vi "Configure Filter.vi"(0 "VISA resource name":refnum<visa-resource-name>, 1 "Scan List (Empty)":string, 5 "Filter Type (0:Off)":u16(ring) items=["Off", "Moving", "Repeat"], 7 "Filter Window (%) (0.1)":dbl=0.1, 9 "Filter Count (10)":i32=10, 11 "error in (no error)":errorcluster) -> (4 "VISA resource name out":refnum<visa-resource-name>, 15 "error out":errorcluster)   [LabVIEW 2020, in "Keithley 27XX.lvlib"]
doc: "This VI configures the filter attributes for the current measurement function.\nFiltering allows you to stabilize noisy measurements. \n\nThe filter setup is \"remembered\" and can be unique for each measurement function. When you change functions , the instrument will return to the last filter setup for that function.\n\nNote: \n(1) Configure Measurement.vi must be called <B>before</B> setting the filter.\n\n(2) This VI should not be used with the measurement functions Frequency, Period, or Continuity."
uses:
  <instrlib>/Keithley 27XX/Keithley 27XX.lvlib
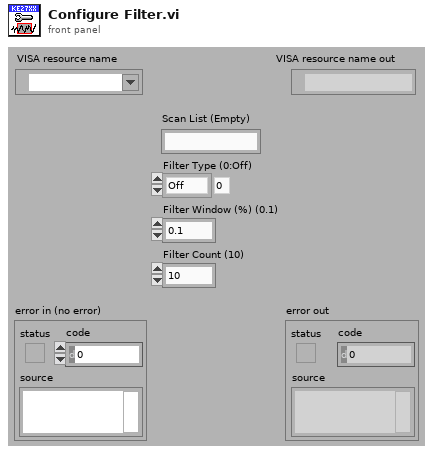
[diagram p1: front panel]
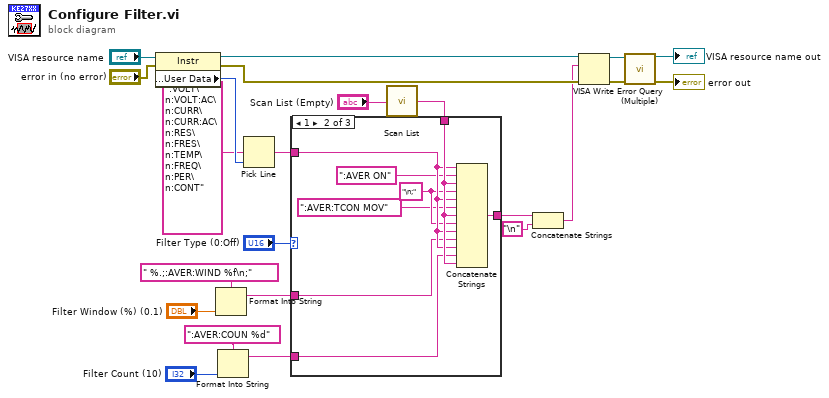
[diagram p0: block diagram]
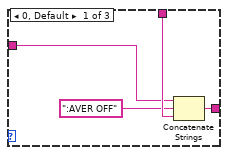
[diagram p2: hidden frame]
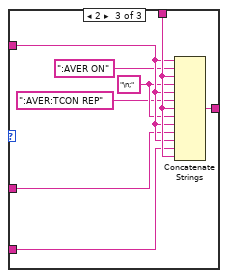
[diagram p3: hidden frame]
diagram:
  n1 = property on="Property Node" class="Instr"(reference="VISA resource name", error in="error in (no error)") -> (reference out=w19:refnum<visa-resource-name>, error out=w18:errorcluster, "General Settings:User Data"=w23:u32)
  n2 = Format Into String(format string=" %.;:AVER:WIND %f\n;", "Filter Window (%) (0.1)") -> (resulting string=w11:string)  [unwired: 2 in, 1 out]
  n3 = Format Into String(format string=":AVER:COUN %d", "Filter Count (10)") -> (resulting string=w9:string)  [unwired: 2 in, 1 out]
  n4 = Pick Line(multi-line string=":VOLT\n:VOLT:AC\n:CURR\n:CURR:AC\n:RES\n:FRES\n:TEMP\n:FREQ\n:PER\n:CONT", line index=w23) -> (output string=w20:string)  [unwired: 1 in]
  n5 = call <instrlib>:"Scan List.vi"("Scan List (Empty)"="Scan List (Empty)") -> ("Scan List Out"=w14:string)  [unwired: 14 in]
  n6 = case shown="1" "Filter Type (0:Off)" {
    tunnel: w20 -> [w25 w33 w41]
    tunnel: w14 -> [w26 w34 w42]
    tunnel: w11 -> [_ w31 w37]
    tunnel: w9 -> [_ w30 w36]
    tunnel: [w27 w35 w43] -> w2
    frame 0, Default {
      n7 = Concatenate Strings(w25, ":AVER OFF", w26) -> (w27:string)
    }
    frame 1 {
      w32 = "\n;" ("string")
      n8 = Concatenate Strings(w33, ":AVER ON", w34, w32, w33, ":AVER:TCON MOV", w34, w32, w33, w31, w33, w30, w34) -> (w35:string)
    }
    frame 2 {
      w39 = "\n;" ("string")
      n9 = Concatenate Strings(w41, ":AVER ON", w42, w39, w41, ":AVER:TCON REP", w42, w39, w41, w37, w41, w36, w42) -> (w43:string)
    }
  }
  n10 = Concatenate Strings(w2, "\n") -> (w1:string)
  n11 = VISA Write(VISA resource name=w19, write buffer=w1, error in (no error)=w18) -> (VISA resource name out=w7:refnum<visa-resource-name>, error out=w6:errorcluster)  [unwired: 1 out]
  n12 = call <instrlib>:"Error Query (Multiple).vi"("VISA resource name"=w7, "error in (no error)"=w6) -> ("VISA resource name out"=→"VISA resource name out":refnum<visa-resource-name>, "error out"=→"error out":errorcluster)  [unwired: 10 in, 2 out]
